vi "Sweep NI-DAQmx Output.vi"(5 "Final Output Value":dbl, 6 "Ramp Rate V/s":dbl=0.04, 7 "Init Input Voltage":dbl=2.009228387670149 format="%0.4f", 8 "error in":errorcluster, 9 "Field Read Voltage":tag="Dev1/ai3", 10 "Output Channel":i32=1, 11 "NI-DAQ Device Number":i32=1) -> (0 "error out":errorcluster)   [LabVIEW 2021]
uses:
  <vilib>/DAQmx/write.llb/DAQmx Write (Analog DBL 1Chan 1Samp).vi
  <vilib>/DAQmx/create/channels.llb/DAQmx Create Channel (AO-Voltage-Basic).vi
  <vilib>/DAQmx/miscellaneous.llb/DAQmx Fill In Error Info.vi
panel:
  out "Voltage applied":dbl format="%^#_4g"
  out "Voltage Read":dbl=0.0026101663032434197 format="%^#_4e"
  out "Delta V":dbl=-2.009228387670149
  out "Number of Steps":i32=1005
  out "Voltage Step Size":dbl=-0.0019992322265374616 format="%^#_6g"
  # "Calculated Sweep Parameters:"
  # "Device Address Parameters:"
  # "Sweep Parameters:"
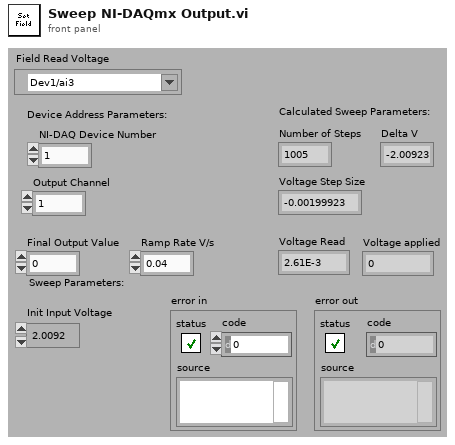
[diagram p1: front panel]
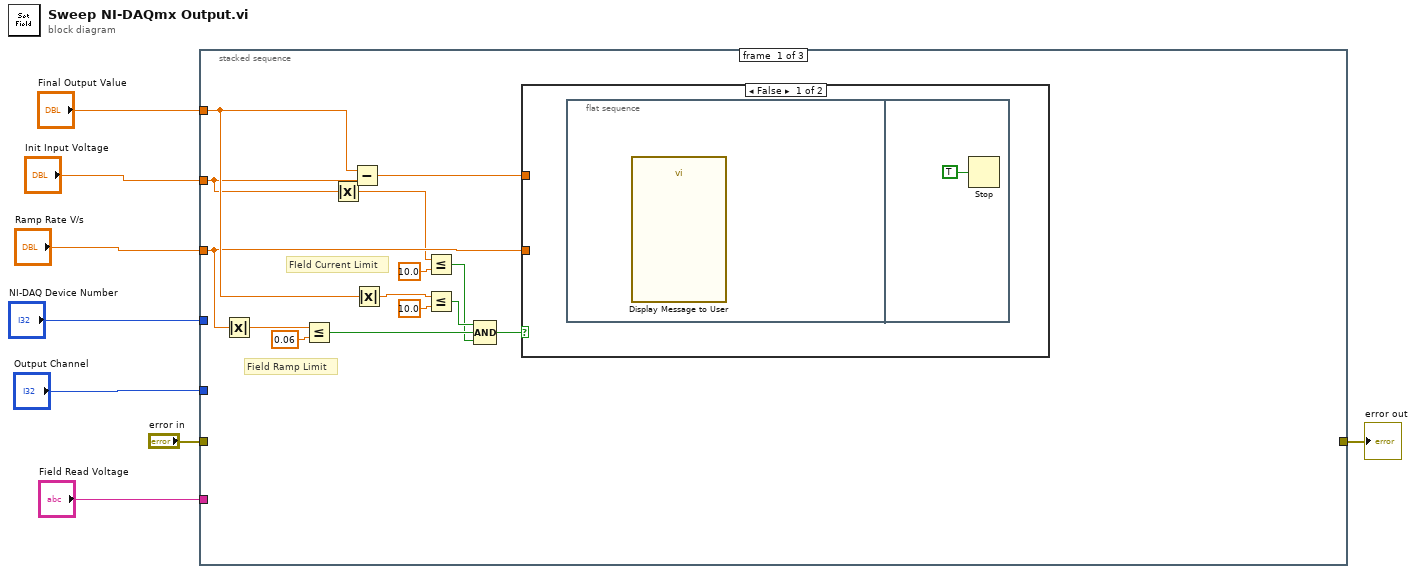
[diagram p0: block diagram]
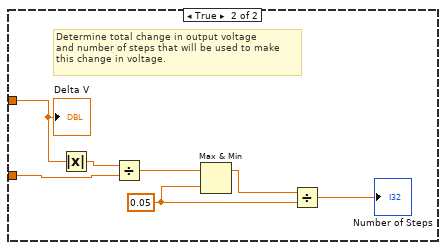
[diagram p2: hidden frame]
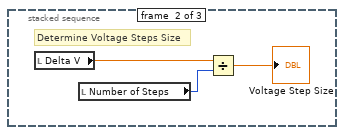
[diagram p3: hidden frame]
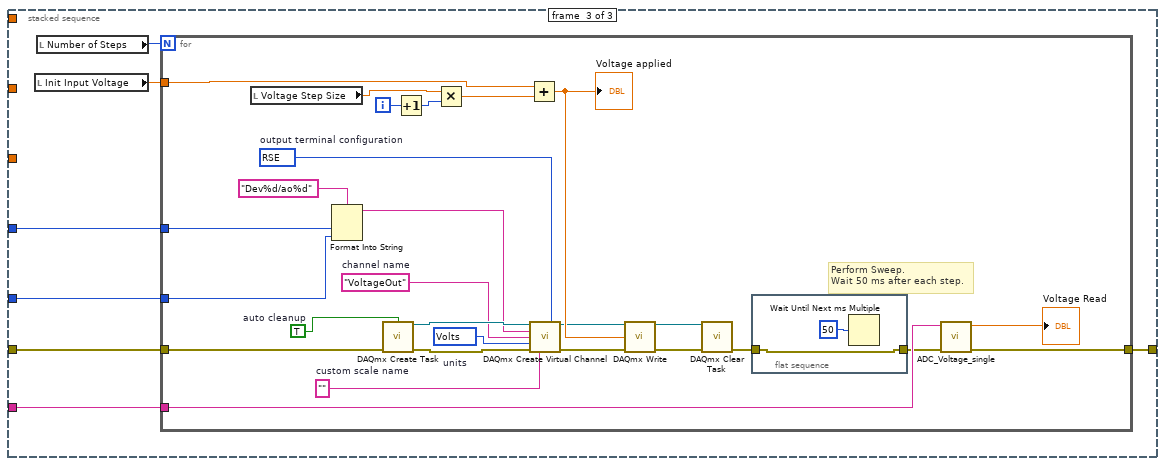
[diagram p4: hidden frame]
diagram:
  n1 = stacked-sequence {
    tunnel: "Final Output Value" -> [w18 _ _]
    tunnel: "Ramp Rate V/s" -> [w15 _ _]
    tunnel: "NI-DAQ Device Number" -> [_ _ w39]
    tunnel: "Output Channel" -> [_ _ w38]
    tunnel: "error in" -> [_ _ w37]
    tunnel: [_ _ w36] -> w3
    tunnel: "Field Read Voltage" -> [_ _ w35]
    tunnel: "Init Input Voltage" -> [w10 _ _]
    frame #0 {
      # "Field Ramp Limit"
      # "FIeld Current Limit"
      n2 = Absolute Value(x=w15) -> (abs(x)=w13:dbl)
      n3 = Less Or Equal?(x=w13, y=0.06) -> (x <= y?=w16:bool)
      n4 = Absolute Value(x=w10) -> (abs(x)=w9:dbl)
      n5 = Subtract(x=w18, y=w10) -> (x-y=w14:dbl)
      n6 = Absolute Value(x=w18) -> (abs(x)=w21:dbl)
      n7 = Less Or Equal?(x=w9, y=10.0) -> (x <= y?=w11:bool)
      n8 = Less Or Equal?(x=w21, y=10.0) -> (x <= y?=w19:bool)
      n9 = Compound Arithmetic op=AND(w19, w16, w11) -> (w20:bool)
      n10 = case shown="False" w20 {
        tunnel: w15 -> [_ w25]
        tunnel: w14 -> [_ w27]
        frame False {
          n11 = flat-sequence {
            frame #0 {
              n12 = call "Display Message to User"() -> ()  [unwired: 10 in, 2 out]
            }
            frame #1 {
              n13 = Stop(stop? (T)=TRUE) -> ()
            }
          }
        }
        frame True {
          w29 = 0.05
          # "Determine total change in output voltage\nand number of steps that will be used to make\nthis change in voltage."
          n14 = Absolute Value(x=w27) -> (abs(x)=w26:dbl)
          n15 = Divide(x=w26, y=w25) -> (x/y=w24:dbl)
          n16 = Max & Min(x=w24, y=w29) -> (max(x,y)=w30:dbl)  [unwired: 1 out]
          n17 = Divide(x=w30, y=w29) -> (x/y=→"Number of Steps":dbl)
          "Delta V" <- w27
        }
      }
    }
    frame #1 {
      # "Determine Voltage Steps Size"
      n18 = local read "Delta V"() -> (w33:dbl)
      n19 = local read "Number of Steps"() -> (w32:i32)
      n20 = Divide(x=w33, y=w32) -> (x/y=→"Voltage Step Size":dbl)
    }
    frame #2 {
      n21 = local read "Init Input Voltage"() -> (w34:dbl)
      n22 = local read "Number of Steps"() -> (w40:i32)
      n23 = for {
        N: w40 -> [_]
        tunnel: w39 -> [w54]
        tunnel: w34 -> [w66]
        tunnel: w38 -> [w53]
        tunnel: w37 -> [w46]
        tunnel: [w42] -> w36
        tunnel: w35 -> [w44]
        i -> [w67]
        w56 = 10083 items=["Default"=-1, "RSE"=10083, "Differential"=10106, "Pseudodifferential"=12529]  # output terminal configuration
        w57 = 10348 items=["Volts"=10348, "From Custom Scale"=10065]  # units
        w58 = "VoltageOut"  # channel name
        w59 = ""  # custom scale name
        w60 = TRUE  # auto cleanup
        # "Perform Sweep.\nWait 50 ms after each step."
        n24 = local read "Voltage Step Size"() -> (w64:dbl)
        n25 = Format Into String(format string="Dev%d/ao%d", w54, w53) -> (resulting string=w52:string)  [unwired: 2 in, 1 out]
        n26 = call <vilib>:"DAQmx Create Task.vi"("auto cleanup"=w60, "error in"=w46) -> ("task out"=w61:refnum<k21>, "error out"=w62:errorcluster)  [unwired: 12 in]
        n27 = Increment(x=w67) -> (x+1=w63:i32)
        n28 = Multiply(x=w64, y=w63) -> (x*y=w65:dbl)
        n29 = Add(x=w66, y=w65) -> (x+y=w49:dbl)
        "Voltage applied" <- w49
        n30 = call-poly <vilib>:"DAQmx Create Virtual Channel.vi"("task in"=w61, "output terminal configuration"=w56, "physical channels"=w52, "name to assign"=w58, "units"=w57, "error in"=w62, "custom scale name"=w59) -> ("task out"=w48:refnum<k21>, "error out"=w47:errorcluster)  [unwired: 7 in]
        n31 = call-poly <vilib>:"DAQmx Write.vi"("task/channels in"=w48, "data"=w49, "error in"=w47) -> ("task out"=w51:refnum<k21>, "error out"=w50:errorcluster)  [unwired: 10 in, 1 out]
        n32 = call <vilib>:"DAQmx Clear Task.vi"("task in"=w51, "error in"=w50) -> ("error out"=w43:errorcluster)  [unwired: 13 in]
        n33 = flat-sequence {
          tunnel: [w69] -> w41
          tunnel: w43 -> [w69]
          frame #0 {
            n34 = Wait Until Next ms Multiple(millisecond multiple=50) -> ()  [unwired: 1 out]
          }
        }
        n35 = call "ADC_Voltage_single.vi"("error in"=w41, "physical channels"=w44) -> ("error out"=w42:errorcluster, "data"=→"Voltage Read":dbl)  [unwired: 8 in]
      }
    }
  }
  "error out" <- w3
